vi "Config.vi"(11 "Config Cluster":T1={"Step Pulse(uS)"=10, "Step Idel Delay(mS)"=25, "Junction Deviation"=0.01, "Arc Tolerance"=0.002, "Homing Feed"=25.0, "Homing Seek"=500.0, "Homing Debounce"=250.0, "Homing Pull-Off"=1.0, "Z Steps"=160.0, "X Max Rate"=1000.0, "Y Max Rate"=1000.0, "Max Spindle "=1000.0, "Z Max Rate"=1000.0, "Min Spindle"=0.0, "X Acceleration"=10.0, "Y Acceleration"=10.0, "X Steps"=160.0, "Y Steps"=160.0, "Z Acceleration"=10.0, "X Max Travel"=1000.0, "Y Max Travel"=600.0, "Z Max Travel"=300.0, "Step Enable Invert"=enum."Disable", "Limit Pins Invert"=enum."Disable", "Status Report"=enum."Postition Type", "Report Unit"=enum."mm", "Probe Pins Invert"=enum."Disable", "Soft Limits"=enum."Enable", "Hard Limits"=enum."Disable", "Homing Cycle"=enum."Enable", "Homing Invert"=enum."X Y Z", "Laser Mode"=enum."OFF", "Step Port Invert"=enum."X Y Z", "Direction Invert"=enum."X' Y' Z'"}) -> (3 "concatenated string":string)   [LabVIEW 2021]
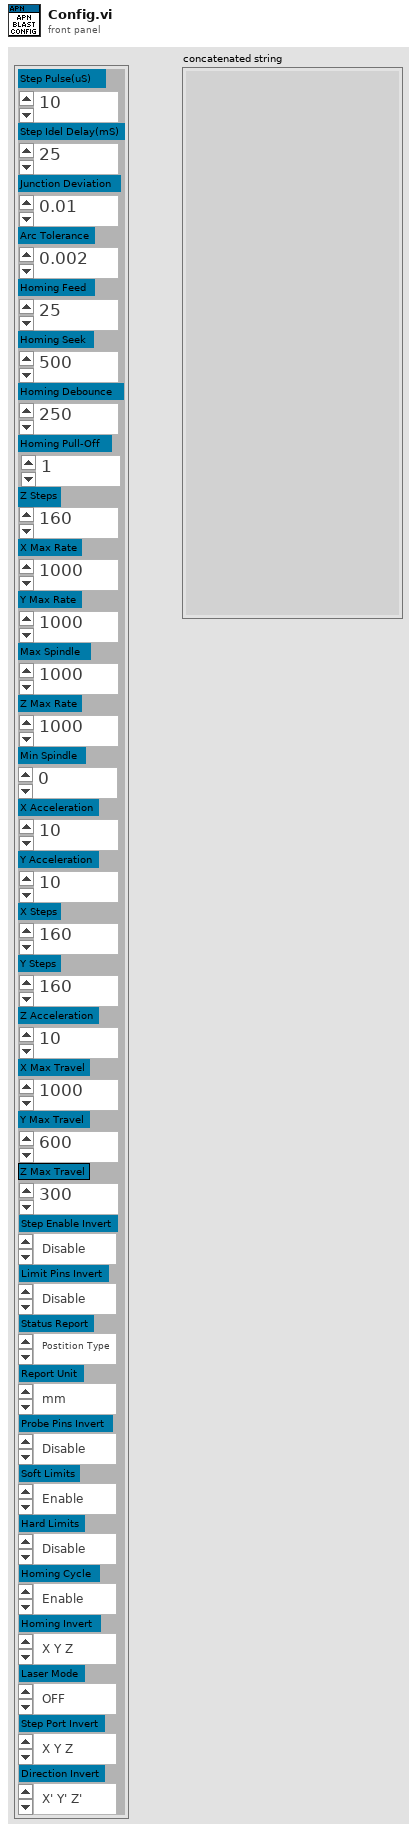
[diagram p1: front panel]
types:
  T1 = cluster{"Step Pulse(uS)":i32, "Step Idel Delay(mS)":i32, "Junction Deviation":dbl, "Arc Tolerance":dbl, "Homing Feed":dbl, "Homing Seek":dbl, "Homing Debounce":dbl, "Homing Pull-Off":dbl, "Z Steps":dbl, "X Max Rate":dbl, "Y Max Rate":dbl, "Max Spindle ":dbl, "Z Max Rate":dbl, "Min Spindle":dbl, "X Acceleration":dbl, "Y Acceleration":dbl, "X Steps":dbl, "Y Steps":dbl, "Z Acceleration":dbl, "X Max Travel":dbl, "Y Max Travel":dbl, "Z Max Travel":dbl, "Step Enable Invert":enum16{"Disable", "Enable"}, "Limit Pins Invert":enum16{"Disable", "Enable"}, "Status Report":enum16{"", "Postition Type", "Buffer Data"}, "Report Unit":enum16{"mm", "Inches"}, "Probe Pins Invert":enum16{"Disable", "Enable"}, "Soft Limits":enum16{"Disable", "Enable"}, "Hard Limits":enum16{"Disable", "Enable"}, "Homing Cycle":enum16{"Disable", "Enable"}, "Homing Invert":enum16{"X Y Z", "X' Y Z", "X Y' Z", "X' Y' Z", "X Y Z'", "X' Y Z'", "X Y' Z'", "X' Y' Z'"}, "Laser Mode":enum16{"OFF", "ON"}, "Step Port Invert":enum16{"X Y Z", "X' Y Z", "X Y' Z", "X' Y' Z", "X Y Z'", "X' Y Z'", "X Y' Z'", "X' Y' Z'"}, "Direction Invert":enum16{"X Y Z", "X' Y Z", "X Y' Z", "X' Y' Z", "X Y Z'", "X' Y Z'", "X Y' Z'", "X' Y' Z'"}}
  T2 = enum16{"X Y Z", "X' Y Z", "X Y' Z", "X' Y' Z", "X Y Z'", "X' Y Z'", "X Y' Z'", "X' Y' Z'"}
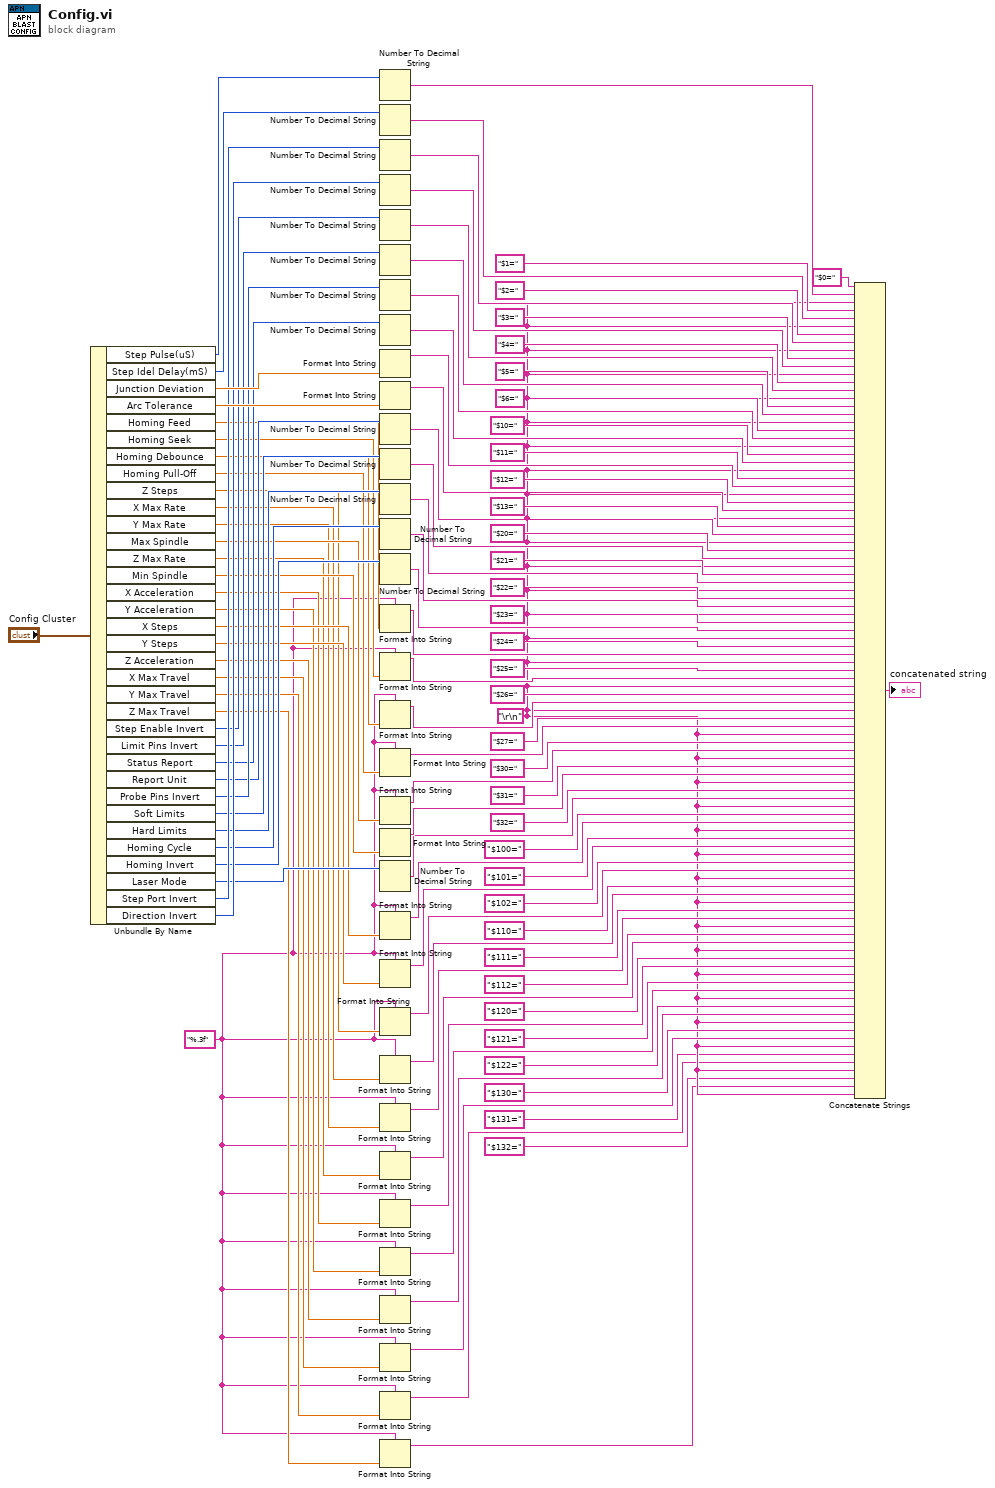
[diagram p0: block diagram]
diagram:
  w2 = "%.3f"
  w7 = "\r\n"
  n1 = Unbundle By Name("Config Cluster") -> ("Step Pulse(uS)"=w81:i32, "Step Idel Delay(mS)"=w80:i32, "Junction Deviation"=w88:dbl, "Arc Tolerance"=w85:dbl, "Homing Feed"=w58:dbl, "Homing Seek"=w56:dbl, "Homing Debounce"=w52:dbl, "Homing Pull-Off"=w50:dbl, "Z Steps"=w32:dbl, "X Max Rate"=w28:dbl, "Y Max Rate"=w26:dbl, "Max Spindle"=w46:dbl, "Z Max Rate"=w23:dbl, "Min Spindle"=w44:dbl, "X Acceleration"=w20:dbl, "Y Acceleration"=w17:dbl, "X Steps"=w38:dbl, "Y Steps"=w35:dbl, "Z Acceleration"=w14:dbl, "X Max Travel"=w12:dbl, "Y Max Travel"=w11:dbl, "Z Max Travel"=w10:dbl, "Step Enable Invert"=w77:enum16{"Disable", "Enable"}, "Limit Pins Invert"=w76:enum16{"Disable", "Enable"}, "Status Report"=w74:enum16{"", "Postition Type", "Buffer Data"}, "Report Unit"=w73:enum16{"mm", "Inches"}, "Probe Pins Invert"=w75:enum16{"Disable", "Enable"}, "Soft Limits"=w71:enum16{"Disable", "Enable"}, "Hard Limits"=w68:enum16{"Disable", "Enable"}, "Homing Cycle"=w64:enum16{"Disable", "Enable"}, "Homing Invert"=w62:T2, "Laser Mode"=w41:enum16{"OFF", "ON"}, "Step Port Invert"=w79:T2, "Direction Invert"=w78:T2)
  n2 = Number To Decimal String(number=w81) -> (decimal integer string=w105:string)  [unwired: 1 in]
  n3 = Number To Decimal String(number=w80) -> (decimal integer string=w103:string)  [unwired: 1 in]
  n4 = Number To Decimal String(number=w79) -> (decimal integer string=w101:string)  [unwired: 1 in]
  n5 = Number To Decimal String(number=w78) -> (decimal integer string=w99:string)  [unwired: 1 in]
  n6 = Number To Decimal String(number=w77) -> (decimal integer string=w97:string)  [unwired: 1 in]
  n7 = Number To Decimal String(number=w76) -> (decimal integer string=w95:string)  [unwired: 1 in]
  n8 = Number To Decimal String(number=w75) -> (decimal integer string=w93:string)  [unwired: 1 in]
  n9 = Number To Decimal String(number=w74) -> (decimal integer string=w90:string)  [unwired: 1 in]
  n10 = Format Into String(w88) -> (resulting string=w87:string)  [unwired: 3 in, 1 out]
  n11 = Format Into String(w85) -> (resulting string=w84:string)  [unwired: 3 in, 1 out]
  n12 = Number To Decimal String(number=w73) -> (decimal integer string=w82:string)  [unwired: 1 in]
  n13 = Number To Decimal String(number=w71) -> (decimal integer string=w70:string)  [unwired: 1 in]
  n14 = Number To Decimal String(number=w68) -> (decimal integer string=w67:string)  [unwired: 1 in]
  n15 = Number To Decimal String(number=w64) -> (decimal integer string=w65:string)  [unwired: 1 in]
  n16 = Number To Decimal String(number=w62) -> (decimal integer string=w61:string)  [unwired: 1 in]
  n17 = Format Into String(format string=w2, w58) -> (resulting string=w59:string)  [unwired: 2 in, 1 out]
  n18 = Format Into String(format string=w2, w56) -> (resulting string=w55:string)  [unwired: 2 in, 1 out]
  n19 = Format Into String(format string=w2, w52) -> (resulting string=w53:string)  [unwired: 2 in, 1 out]
  n20 = Format Into String(format string=w2, w50) -> (resulting string=w49:string)  [unwired: 2 in, 1 out]
  n21 = Format Into String(format string=w2, w46) -> (resulting string=w47:string)  [unwired: 2 in, 1 out]
  n22 = Format Into String(w44) -> (resulting string=w43:string)  [unwired: 3 in, 1 out]
  n23 = Number To Decimal String(number=w41) -> (decimal integer string=w40:string)  [unwired: 1 in]
  n24 = Format Into String(format string=w2, w38) -> (resulting string=w37:string)  [unwired: 2 in, 1 out]
  n25 = Format Into String(format string=w2, w35) -> (resulting string=w34:string)  [unwired: 2 in, 1 out]
  n26 = Format Into String(format string=w2, w32) -> (resulting string=w31:string)  [unwired: 2 in, 1 out]
  n27 = Format Into String(format string=w2, w28) -> (resulting string=w29:string)  [unwired: 2 in, 1 out]
  n28 = Format Into String(format string=w2, w26) -> (resulting string=w25:string)  [unwired: 2 in, 1 out]
  n29 = Format Into String(format string=w2, w23) -> (resulting string=w22:string)  [unwired: 2 in, 1 out]
  n30 = Format Into String(format string=w2, w20) -> (resulting string=w19:string)  [unwired: 2 in, 1 out]
  n31 = Format Into String(format string=w2, w17) -> (resulting string=w16:string)  [unwired: 2 in, 1 out]
  n32 = Format Into String(format string=w2, w14) -> (resulting string=w13:string)  [unwired: 2 in, 1 out]
  n33 = Format Into String(format string=w2, w12) -> (resulting string=w8:string)  [unwired: 2 in, 1 out]
  n34 = Format Into String(format string=w2, w11) -> (resulting string=w4:string)  [unwired: 2 in, 1 out]
  n35 = Format Into String(format string=w2, w10) -> (resulting string=w3:string)  [unwired: 2 in, 1 out]
  n36 = Concatenate Strings("$0=", w105, w7, "$1=", w103, w7, "$2=", w101, w7, "$3=", w99, w7, "$4=", w97, w7, "$5=", w95, w7, "$6=", w93, w7, "$10=", w90, w7, "$11=", w87, w7, "$12=", w84, w7, "$13=", w82, w7, "$20=", w70, w7, "$21=", w67, w7, "$22=", w65, w7, "$23=", w61, w7, "$24=", w59, w7, "$25=", w55, w7, "$26=", w53, w7, "$27=", w49, w7, "$30=", w47, w7, "$31=", w43, w7, "$32=", w40, w7, "$100=", w37, w7, "$101=", w34, w7, "$102=", w31, w7, "$110=", w29, w7, "$111=", w25, w7, "$112=", w22, w7, "$120=", w19, w7, "$121=", w16, w7, "$122=", w13, w7, "$130=", w8, w7, "$131=", w4, w7, "$132=", w3, w7) -> (→"concatenated string":string)
